vi "createBehParaArray.vi"(1 "ParaCluster":T1) -> (0 "behParaArray":sgl[](array[numeric]))   [LabVIEW 2014]
uses:
  ParaCluster_def.ctl
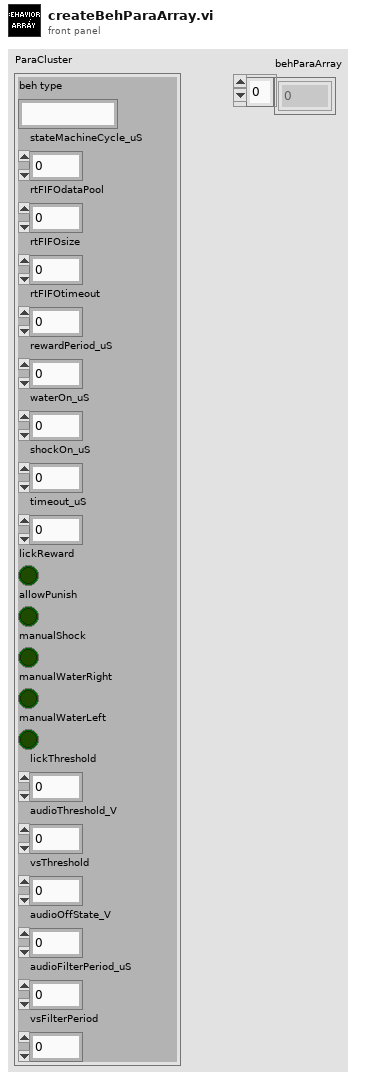
[diagram p1: front panel]
types:
  T1 = typedef "ParaCluster_def.ctl" = cluster{"beh type":string, "stateMachineCycle_uS":u32, "rtFIFOdataPool":u32, "rtFIFOsize":u32, "rtFIFOtimeout":u32, "rewardPeriod_uS":u32, "waterOn_uS":u32, "shockOn_uS":u32, "timeout_uS":u32, "lickReward":bool, "allowPunish":bool, "manualShock":bool, "manualWaterRight":bool, "manualWaterLeft":bool, "lickThreshold":fxp<+/-,16,5>, "audioThreshold_V":fxp<+/-,16,5>, "vsThreshold":fxp<+/-,16,5>, "audioOffState_V":fxp<+/-,16,5>, "audioFilterPeriod_uS":i32, "vsFilterPeriod":i32}
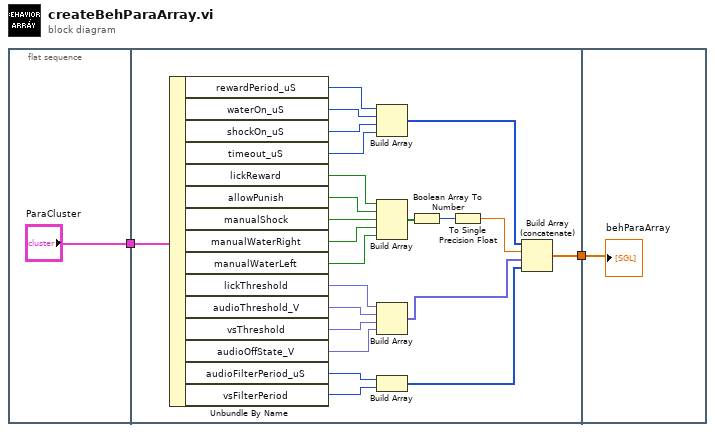
[diagram p0: block diagram]
diagram:
  n1 = flat-sequence {
    tunnel: ["ParaCluster"] -> w1
    tunnel: [w5] -> w2
    tunnel: w1 -> [w4]
    tunnel: w2 -> [w27]
    frame #0 {
    }
    frame #1 {
      n2 = Unbundle By Name(w4) -> ("rewardPeriod_uS"=w26:u32, "waterOn_uS"=w25:u32, "shockOn_uS"=w24:u32, "timeout_uS"=w23:u32, "lickReward"=w22:bool, "allowPunish"=w21:bool, "manualShock"=w20:bool, "manualWaterRight"=w19:bool, "manualWaterLeft"=w18:bool, "lickThreshold"=w17:fxp<+/-,16,5>, "audioThreshold_V"=w16:fxp<+/-,16,5>, "vsThreshold"=w15:fxp<+/-,16,5>, "audioOffState_V"=w14:fxp<+/-,16,5>, "audioFilterPeriod_uS"=w13:i32, "vsFilterPeriod"=w12:i32)
      n3 = Build Array(w26, w25, w24, w23) -> (w9:u32[])
      n4 = Build Array ("para")(w22, w21, w20, w19, w18) -> (w11:bool[])
      n5 = Build Array ("para")(w17, w16, w15, w14) -> (w7:fxp<+/-,16,5>[])
      n6 = Build Array ("para")(w13, w12) -> (w6:i32[])
      n7 = Boolean Array To Number(Boolean array=w11) -> (number=w10:u32)
      n8 = To Single Precision Float(number=w10) -> (single precision float=w8:sgl)
      n9 = Build Array (concatenate)(w9, w8, w7, w6) -> (w5:sgl[])
    }
    frame #2 {
      "behParaArray" <- w27
    }
  }
